vi "configure operation.vi"(7 "CVT configuration":refnum<class "TEC configuration.lvclass">, 8 "error in":errorcluster, 10 "line item in":T1, 11 "engine configuration in":refnum<class "engine configuration.lvclass">) -> (0 "error out":errorcluster, 1 "success":bool, 2 "line item out":T1, 5 "changed":bool)   [LabVIEW 2013, in "TEC editor node.lvclass"]
uses:
  TEC editor node.lvclass
  permissions.ctl
  <vilib>/NI/Tag Bus/tag/Data Type.ctl
  table line.ctl
  <vilib>/NI/Tag Bus Module Framework/channel/TBM channel.lvclass
  <vilib>/NI/Module Execution Interface/Engine Configuration/engine configuration.lvclass
  module/configuration/TEC configuration.lvclass
  <vilib>/NI/Tag Bus Module Framework/root configuration/TBM configuration.lvclass/TBM configuration.ctl
  <vilib>/NI/Tag Bus Module Framework/channel/TBM channel.lvclass/TBM channel.ctl
  <vilib>/NI/Tag Bus/tag/tag descriptor.lvclass/tag descriptor.ctl
  <vilib>/NI/Tag Bus Module Framework/channel/Read channel classification.vi
  <vilib>/NI/Tag Bus/tag/read data type.vi
  <vilib>/NI/Tag Bus/tag/write tag name.vi
  <vilib>/NI/Tag Bus/tag/write data type.vi
  <vilib>/NI/Tag Bus Module Framework/channel/Write channel classification.vi
  <vilib>/NI/Tag Bus Module Framework/root configuration/create GUID.vi
  <vilib>/NI/Tag Bus/tag/tag descriptor.lvclass
  <vilib>/NI/Tag Bus Module Framework/root configuration/TBM configuration.lvclass
panel:
  out "issues":string
  in  "Linked Tag":u16(ring) items=["", "mydouble", "mydouble2"]
  in  "TEC Tag Name":string
  in  "cancel":bool
  in  "ok":bool
  in  "Data Type":T2=enum."Single"
  in  "Access Type":T3
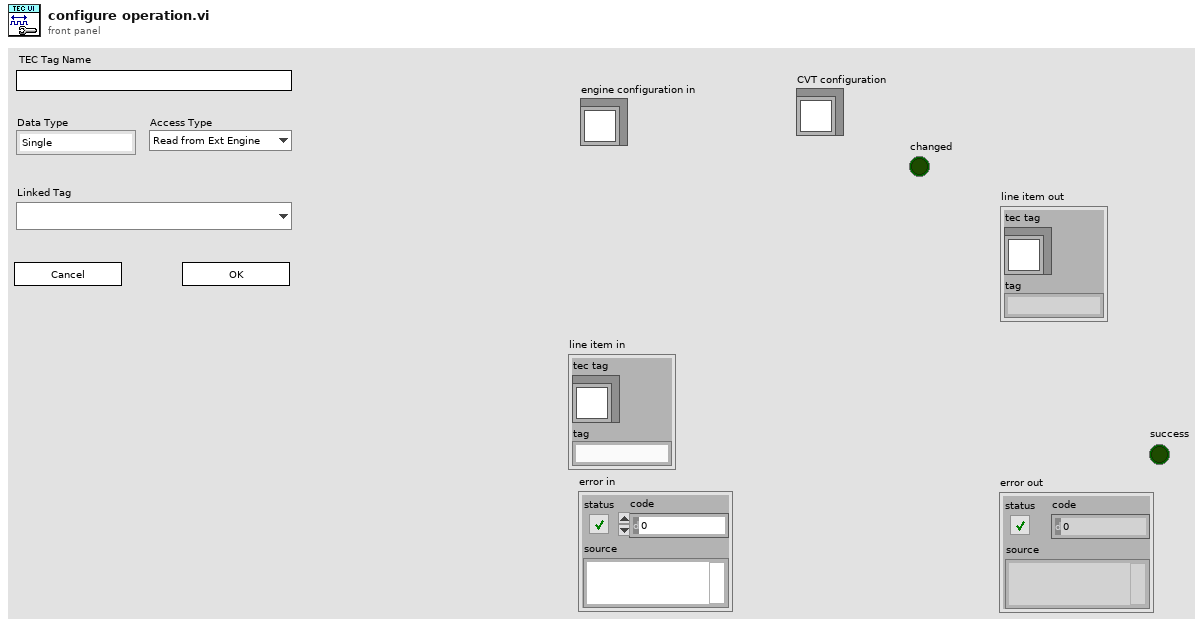
[diagram p1: front panel]
types:
  T1 = typedef "TEC editor node.lvclass/table line.ctl" = cluster{"tec tag":refnum<class "TBM channel.lvclass">, "tag":string}
  T2 = typedef "tag bus.lvlib/tag descriptor.lvclass/Data Type.ctl" = enum16{"Double", "Single", "I64", "I32", "I16", "I8", "U64", "U32", "U16", "U8", "Boolean", "String", "Array of Double", "Array of Single", "Array of I64", "Array of I32", "Array of I16", "Array of I8", "Array of U64", "Array of U32", "Array of U16", "Array of U8", "Array of Boolean", "Array of String"}
  T3 = typedef "TEC editor node.lvclass/permissions.ctl" = enum16{"Read from Ext Engine", "Write to Ext Engine"}
  T4 = enum32{"Invalid", "Standard", "Closed", "Hidden", "Minimized", "Maximized"}
  T5 = enum32{"Invalid", "Default", "Floating", "Floating/Auto-Hide", "Modal"}
  T6 = enum8{"Enabled", "Disabled", "Disabled and Grayed Out"}
  T7 = enum32{"invalid app kind", "Development System", "Run Time System", "Student Edition", "Embedded LabVIEW", "Evaluation", "Custom"}
  T8 = typedef "TBM channel.lvclass/channel classification.ctl" = enum16{"input data", "output data", "processing parameter", "processing result"}
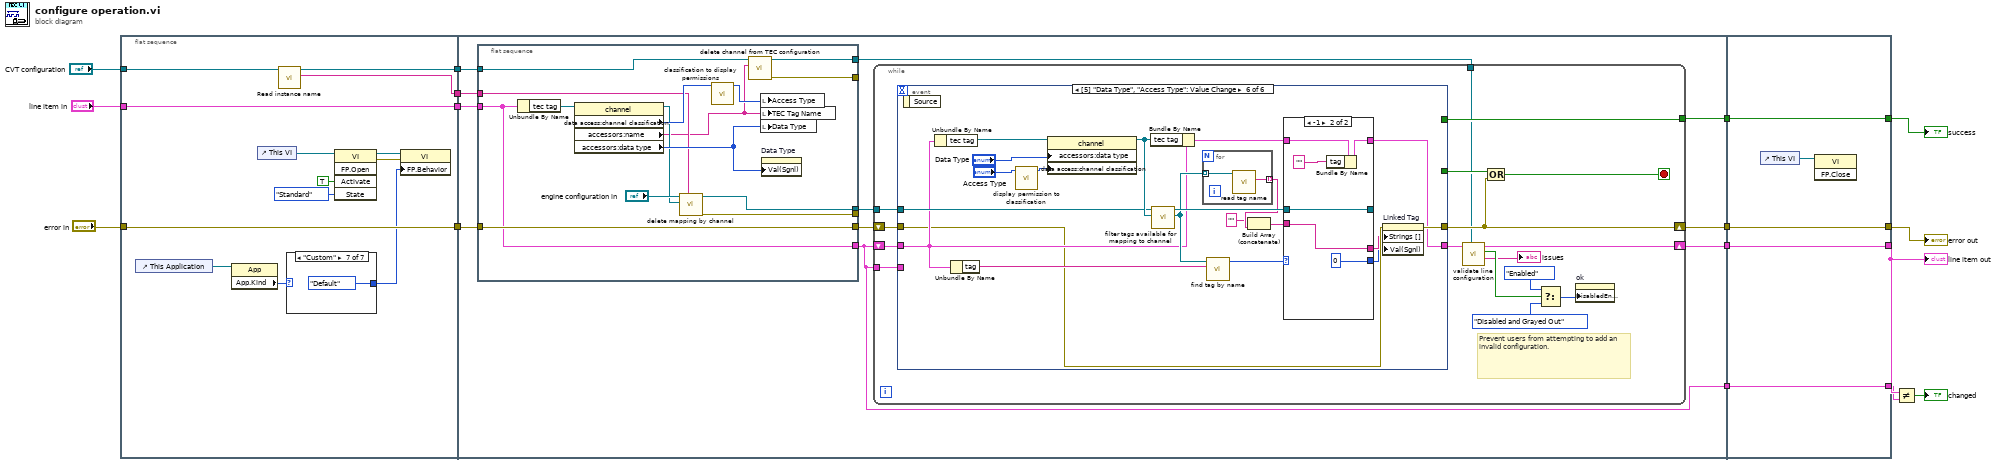
[diagram p0: block diagram]
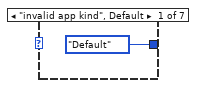
[diagram p2: hidden frame]
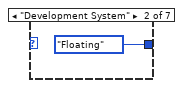
[diagram p3: hidden frame]
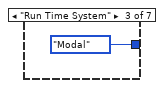
[diagram p4: hidden frame]
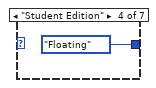
[diagram p5: hidden frame]
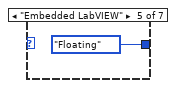
[diagram p6: hidden frame]
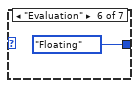
[diagram p7: hidden frame]
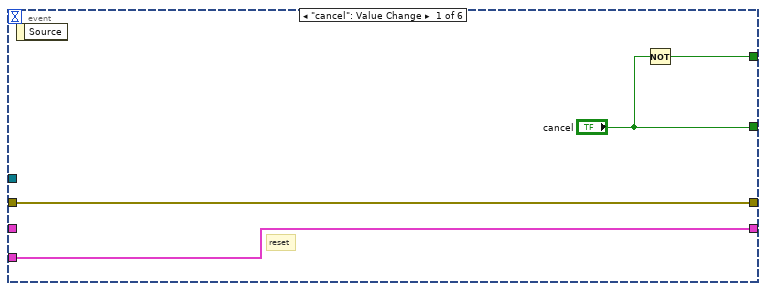
[diagram p8: hidden frame]
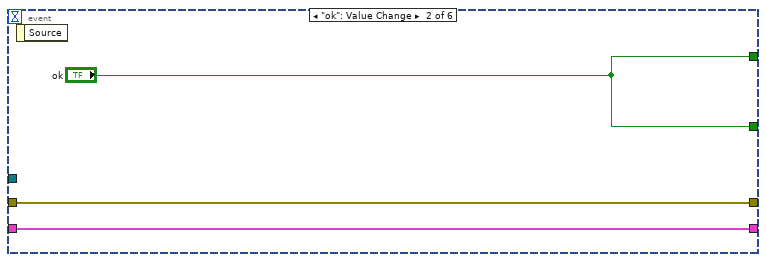
[diagram p9: hidden frame]
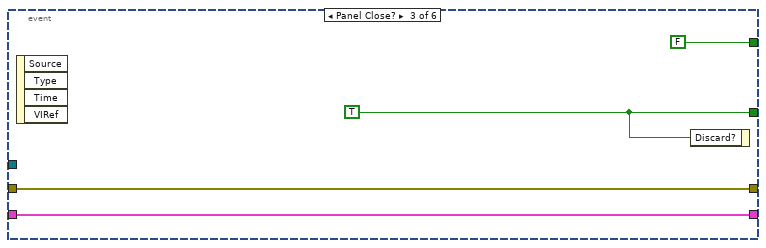
[diagram p10: hidden frame]
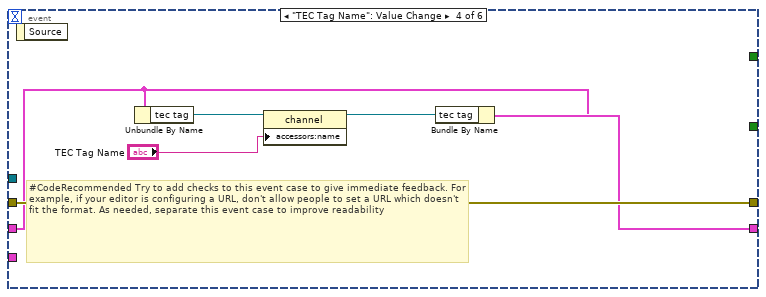
[diagram p11: hidden frame]
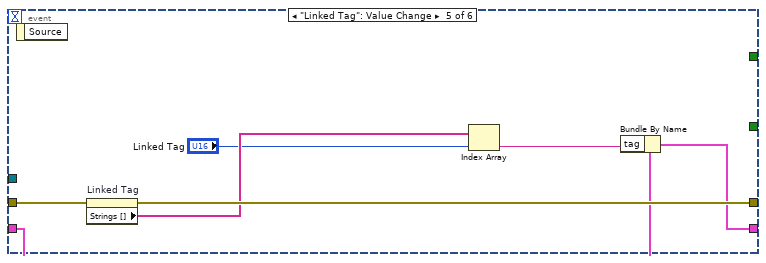
[diagram p12: hidden frame]
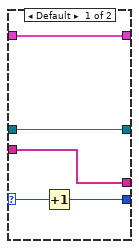
[diagram p13: hidden frame]
diagram:
  n1 = flat-sequence {
    tunnel: "line item in" -> [w28]
    tunnel: "error in" -> [w29]
    tunnel: [w29] -> w5
    tunnel: [w28] -> w4
    tunnel: [w18] -> w3
    tunnel: "CVT configuration" -> [w19]
    tunnel: [w17] -> w1
    tunnel: [w44] -> w9
    tunnel: [w43] -> w8
    tunnel: [w42] -> w7
    tunnel: [w40] -> w6
    tunnel: w5 -> [w47]
    tunnel: w4 -> [w41]
    tunnel: w3 -> [w38]
    tunnel: w1 -> [w39]
    tunnel: [w137] -> w10
    tunnel: [w138] -> w13
    tunnel: [w139] -> w14
    tunnel: [w140] -> w15
    tunnel: w9 -> [w140]
    tunnel: w8 -> [w139]
    tunnel: w7 -> [w138]
    tunnel: w6 -> [w137]
    frame #0 {
      n2 = control-ref of="This Application"() -> (w22:refnum<vi>)
      n3 = property class="App"(reference=w22) -> ("App.Kind"=w21:T7)  [unwired: 1 in, 2 out]
      n4 = control-ref of="This VI"() -> (w23:refnum<vi>)
      n5 = call <vilib>:"Read instance name.vi"("configuration in"=w19) -> ("instance id"=w17:string, "configuration out"=w18:refnum<class "TEC configuration.lvclass">)  [unwired: 8 in, 1 out]
      n6 = case shown="\"Custom\"" w21 {
        tunnel: [T5."Default" ("Front Panel Window:Behavior") T5."Floating" ("Front Panel Window:Behavior") T5."Modal" ("Front Panel Window:Behavior") T5."Floating" ("Front Panel Window:Behavior") T5."Floating" ("Front Panel Window:Behavior") T5."Floating" ("Front Panel Window:Behavior") T5."Default" ("Front Panel Window:Behavior")] -> w20
        frame "invalid app kind", Default {
        }
        frame "Development System" {
        }
        frame "Run Time System" {
        }
        frame "Student Edition" {
        }
        frame "Embedded LabVIEW" {
        }
        frame "Evaluation" {
        }
        frame "Custom" {
        }
      }
      n7 = invoke class="VI" method="FP.Open"(reference=w23, "Activate"=TRUE ("Activate?"), "State"=T4."Standard") -> (reference out=w26:refnum<vi>, error out=w27:errorcluster)  [unwired: 2 in, 3 out]
      n8 = property class="VI"(reference=w26, error in=w27, "FP.Behavior"=w20) -> ()  [unwired: 2 out]
    }
    frame #1 {
      n9 = flat-sequence {
        tunnel: [w135] -> w45
        tunnel: w47 -> [w135]
        tunnel: [w128] -> w46
        tunnel: w41 -> [w134]
        tunnel: [w134] -> w40
        tunnel: w39 -> [w127]
        tunnel: [w126] -> _
        tunnel: w38 -> [w125]
        tunnel: [w123] -> _
        tunnel: [w122] -> w37
        frame #0 {
          n10 = Unbundle By Name(w134) -> ("tec tag"=w132:refnum<class "TBM channel.lvclass">)
          n11 = property class="channel"(reference=w132) -> (reference out=w124:refnum<class "TBM channel.lvclass">, "data access:channel classification"=w130:T8, "accessors:name"=w121:string, "accessors:data type"=w131:T2)  [unwired: 1 in, 1 out]
          n12 = call <vilib>:"delete mapping by channel.vi"("owner ID"=w127, "channel"=w124, "engine configuration in"="engine configuration in") -> ("error out"=w126:errorcluster, "engine configuration out"=w128:refnum<class "engine configuration.lvclass">)  [unwired: 7 in]
          n13 = call "classification to display permissions.vi"("channel classification"=w130) -> ("permissions"=w133:T3)  [unwired: 10 in]
          n14 = call "delete channel from TEC configuration.vi"("channel to delete"=w121, "TEC configuration in"=w125) -> ("error out"=w123:errorcluster, "TEC configuration out"=w122:refnum<class "TEC configuration.lvclass">)  [unwired: 8 in]
          n15 = local write "Access Type"(w133) -> ()
          n16 = local write "TEC Tag Name"(w121) -> ()
          n17 = local write "Data Type"(w131) -> ()
          n18 = property on="Data Type" class="Enum (strict)"("Val(Sgnl)"=w131) -> ()  [unwired: 2 in, 2 out]
        }
      }
      n19 = while {
        shift-right: [w59] -> w43
        shift-left: w45 -> [w62]
        tunnel: [w61] -> w44
        shift-right: [w50] -> w42
        shift-left: w40 -> [w57]
        tunnel: w40 -> [w56]
        tunnel: w46 -> [w63]
        tunnel: w37 -> [w49]
        stop <- w58 stop-if-true
        # "Prevent users from attempting to add an invalid configuration."
        n20 = event shown="[5] \"Data Type\", \"Access Type\": Value Change" {
          selector: _ -> [_ _ _ _ _ _]
          dyn-events: _ -> [_ _ _ _ _ _]
          timeout: _ -> [_ _ _ _ _ _]
          tunnel: w63 -> [_ _ _ _ _ w97]
          tunnel: w62 -> [w67 w69 w74 w80 w87 w95]
          tunnel: [w67 w69 w74 w80 w86 w107] -> w59
          tunnel: [w66 "ok" FALSE _ _ _] -> w61
          tunnel: ["cancel" "ok" w72 _ _ _] -> w60
          tunnel: w57 -> [_ w68 w71 w78 w83 w96]
          tunnel: [w64 w68 w71 w79 w81 w92] -> w51
          tunnel: w56 -> [w64 _ _ _ _ _]
          event "cancel": Value Change {
            # "reset"
            n21 = event-data() -> ()  [unwired: 1 in, 1 out]
            n22 = Not(x="cancel") -> (.not. x?=w66:bool)
          }
          event "ok": Value Change {
            n23 = event-data() -> ()  [unwired: 1 in, 1 out]
          }
          event Panel Close? {
            w72 = TRUE ("cancel")
            n24 = event-data() -> ()  [unwired: 1 in, 4 out]
            n25 = event-data("Discard?"=w72) -> ()  [unwired: 1 in, 1 out]
          }
          event "TEC Tag Name": Value Change {
            # "#CodeRecommended Try to add checks to this event case to give immediate feedback. For example, if your editor is configuring a URL, don't allow people to set a URL which doesn't fit the format. As needed, separate this event case to improve readability"
            n26 = event-data() -> ()  [unwired: 1 in, 1 out]
            n27 = Unbundle By Name(w78) -> ("tec tag"=w77:refnum<class "TBM channel.lvclass">)
            n28 = property class="channel"(reference=w77, "accessors:name"="TEC Tag Name") -> (reference out=w76:refnum<class "TBM channel.lvclass">)  [unwired: 1 in, 1 out]
            n29 = Bundle By Name(cluster=w78, "tec tag"=w76) -> (w79:T1)
          }
          event "Linked Tag": Value Change {
            n30 = event-data() -> ()  [unwired: 1 in, 1 out]
            n31 = property on="Linked Tag" class="Ring (strict)"(error in=w87) -> (error out=w86:errorcluster, "Strings []"=w85:string[])  [unwired: 1 in, 1 out]
            n32 = Index Array(array=w85, index="Linked Tag") -> (element=w82:string)
            n33 = Bundle By Name(cluster=w83, "tag"=w82) -> (w81:T1)
          }
          event Value Change {
            n34 = event-data() -> ()  [unwired: 1 in, 1 out]
            n35 = Unbundle By Name(w96) -> ("tec tag"=w106:refnum<class "TBM channel.lvclass">)
            n36 = Unbundle By Name(w96) -> ("tag"=w104:string)
            n37 = call "display permission to classification.vi"("display permissions"="Access Type") -> ("channel classification"=w89:T8)  [unwired: 10 in]
            n38 = property class="channel"(reference=w106, "accessors:data type"="Data Type", "data access:channel classification"=w89) -> (reference out=w105:refnum<class "TBM channel.lvclass">)  [unwired: 1 in, 1 out]
            n39 = Bundle By Name(cluster=w96, "tec tag"=w105) -> (w103:T1)
            n40 = call <vilib>:"filter tags available for mapping to channel.vi"("channel to map to"=w105, "engine configuration in"=w97) -> ("filtered tags"=w100:refnum<class "tag descriptor.lvclass">[], "engine configuration out"=w102:refnum<class "engine configuration.lvclass">)  [unwired: 8 in]
            n41 = for {
              tunnel: w100 -> [w109] mode=indexing
              tunnel: [w108] -> w99 mode=indexing
              n42 = call <vilib>:"read tag name.vi"("system tag in"=w109) -> ("name"=w108:string)  [unwired: 8 in, 2 out]
            }
            n43 = call <vilib>:"find tag by name.vi"("name"=w104, "tags in"=w100) -> ("index"=w101:i32)  [unwired: 9 in]
            n44 = Build Array (concatenate)("", w99) -> (w88:string[])
            n45 = case shown="-1" w101 {
              selector: w101 -> [w112 _]
              tunnel: [w111 w115] -> w94
              tunnel: [w110 0 ("index")] -> w93
              tunnel: w103 -> [w114 w120]
              tunnel: [w114 w119] -> w92
              tunnel: w102 -> [w113 w117]
              tunnel: [w113 w117] -> _
              tunnel: w88 -> [w111 w115]
              frame Default {
                n46 = Increment(x=w112) -> (x+1=w110:i32)
              }
              frame -1 {
                n47 = Bundle By Name(cluster=w120, "tag"="") -> (w119:T1)
              }
            }
            n48 = property on="Linked Tag" class="Ring (strict)"(error in=w95, "Strings []"=w94, "Val(Sgnl)"=w93) -> (error out=w107:errorcluster)  [unwired: 1 in, 1 out]
          }
        }
        n49 = call "validate line configuration.vi"("TEC configuration"=w49, "line in"=w51) -> ("error"=→"issues":string, "valid?"=w55:bool, "line out"=w50:T1)  [unwired: 7 in]
        n50 = Compound Arithmetic op=OR(w60, w59) -> (w58:bool)
        n51 = Select(t=T6."Enabled" ("Disabled"), s=w55, f=T6."Disabled and Grayed Out") -> (s? t:f=w52:T6)
        n52 = property on="ok" class="Bool"("DisabledEnum"=w52) -> ()  [unwired: 2 in, 2 out]
      }
    }
    frame #2 {
      n53 = control-ref of="This VI"() -> (w136:refnum<vi>)
      n54 = invoke class="VI" method="FP.Close"(reference=w136) -> ()  [unwired: 2 in, 3 out]
    }
  }
  n55 = Not Equal?(x=w13, y=w10) -> (x != y?=→"changed":bool)
  "error out" <- w14
  "success" <- w15
  "line item out" <- w13
